vi "Example Write File - Check Error.vi"(8 "error code":u8, 11 "error in":errorcluster) -> (3 "error out":errorcluster)   [LabVIEW 2010]
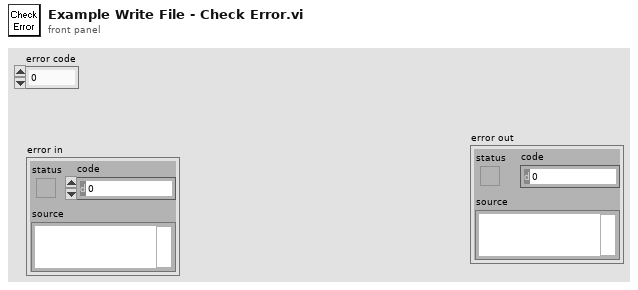
[diagram p1: front panel]
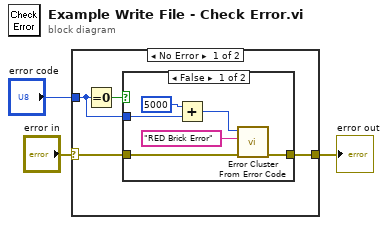
[diagram p0: block diagram]
diagram:
  n1 = case shown="No Error" "error in" {
    selector: "error in" -> [w5 w15]
    tunnel: [w6 w15] -> w2
    tunnel: "error code" -> [w4 _]
    frame No Error {
      n2 = Equal To 0?(x=w4) -> (x = 0?=w7:bool)
      n3 = case shown="False" w7 {
        tunnel: [w13 w14] -> w6
        tunnel: w5 -> [w12 w14]
        tunnel: w4 -> [w10 _]
        frame False {
          n4 = Add(x=5000, y=w10) -> (x+y=w9:i32)
          n5 = call <vilib>:"Error Cluster From Error Code.vi"("error in (no error)"=w12, "error message (\"\")"="RED Brick Error" ("error message (\"\")"), "error code (0)"=w9) -> ("error out"=w13:errorcluster)  [unwired: 6 in]
        }
        frame True {
          # "Success"
        }
      }
    }
    frame Error {
    }
  }
  "error out" <- w2
